vi "Output Select.vi"(8 "error in (no error)":errorcluster, 9 "Instrument Select (Output 1)":string(combo)="OUT1", 11 "VISA resource name":refnum<visa-resource-name>) -> (0 "error out":errorcluster, 3 "VISA resource name out":refnum<visa-resource-name>)   [LabVIEW 2013]
doc: "Selects the output to be configured.\n\nNotes:\n\n(1) Only one output may be selected at a time. Any configuration made to the current output does not affect the other output in anyway.\n\n(2) This VI ONLY applies to models E3646A, E3647A, E3648A, & E3649A"
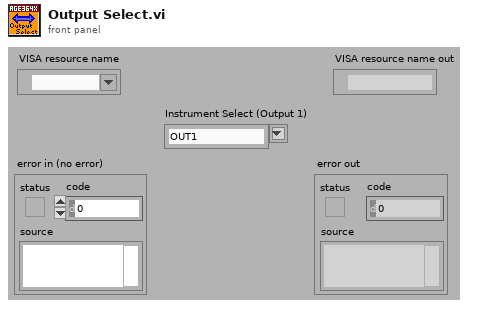
[diagram p1: front panel]
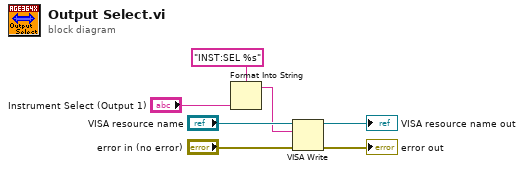
[diagram p0: block diagram]
diagram:
  n1 = Format Into String(format string="INST:SEL %s", "Instrument Select (Output 1)") -> (resulting string=w1:string)  [unwired: 2 in, 1 out]
  n2 = VISA Write(VISA resource name="VISA resource name", write buffer=w1, error in (no error)="error in (no error)") -> (VISA resource name out=→"VISA resource name out":refnum<visa-resource-name>, error out=→"error out":errorcluster)  [unwired: 1 out]
